vi "ETCS_decodeur.vi"(0 "chaine entree":string) -> (1 "Args":dbl[](array[numeric]) format="%.8f", 2 "nb args":i32, 3 "OK done":bool)   [LabVIEW 2011]
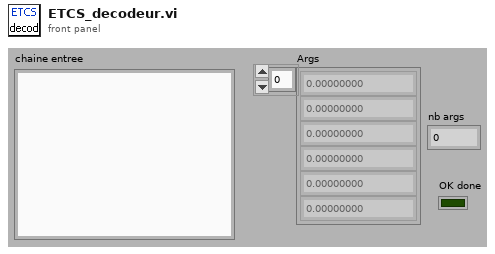
[diagram p1: front panel]
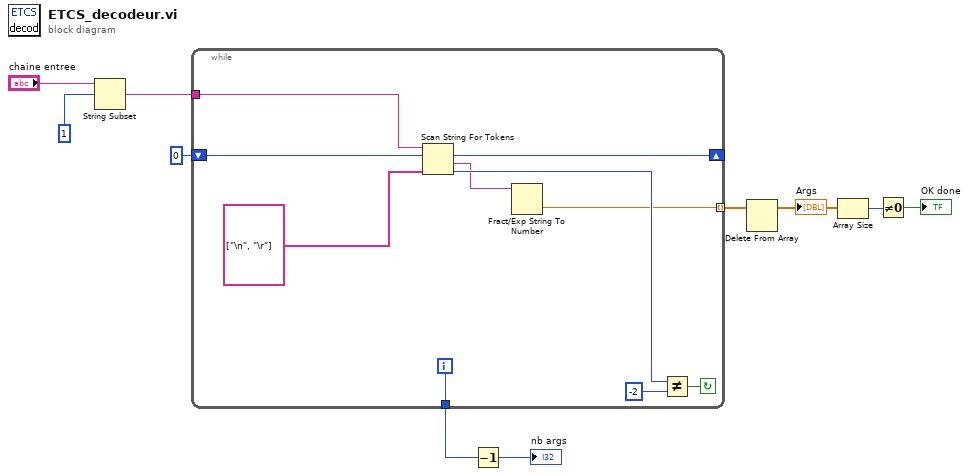
[diagram p0: block diagram]
diagram:
  n1 = String Subset(string="chaine entree", offset (0)=1) -> (substring=w2:string)  [unwired: 1 in]
  n2 = while {
    shift-right: [w14] -> _
    shift-left: 0 ("offset past token") -> [w16]
    tunnel: [w15] -> w9
    tunnel: [w13] -> w8 mode=indexing
    tunnel: w2 -> [w11]
    i -> [w15]
    stop <- w19 continue-if-true
    n3 = Scan String For Tokens(6:string[] ["\n", "\r"] ("delimiters (\\s,\\t,\\r,\\n)"), 8:w16, 9:w11) -> (0:w17:i32, 1:w12:string, 2:w14:i32)  [unwired: 3 in, 1 out]
    n4 = Fract/Exp String To Number(string=w12) -> (number=w13:dbl)  [unwired: 3 in, 1 out]
    n5 = Not Equal?(x=w17, y=-2) -> (x != y?=w19:bool)
  }
  n6 = Decrement(x=w9) -> (x-1=→"nb args":i32)
  n7 = Delete From Array(array=w8) -> (array with subset deleted=w7:dbl[])  [unwired: 2 in, 1 out]
  "Args" <- w7
  n8 = Array Size(array=w7) -> (size(s)=w6:i32)
  n9 = Not Equal To 0?(x=w6) -> (x != 0?=→"OK done":bool)
